vi "Get GEA3 COM Port.vi"(0 "GEA3 Serial Number":string, 11 "Error In":errorcluster) -> (4 "GEA3 COM Port":string, 15 "Error Out":errorcluster)   [LabVIEW 2016, in "GEA2_Toolkit.lvlib"]
uses:
  library/GEA2_Toolkit.lvlib
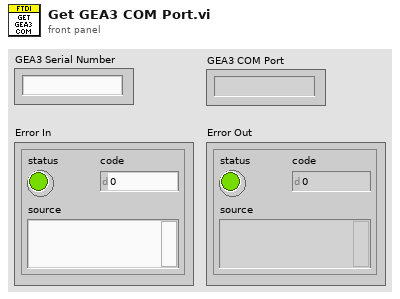
[diagram p1: front panel]
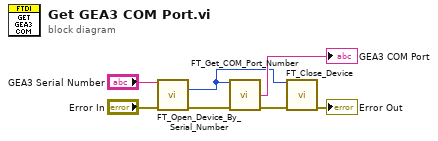
[diagram p0: block diagram]
diagram:
  n1 = call "FT_Open_Device_By_Serial_Number.vi"("Device Serial Number"="GEA3 Serial Number", "Error In"="Error In") -> ("Handle"=w4:u32, "Error Out"=w3:errorcluster)  [unwired: 11 in, 1 out]
  n2 = call "FT_Get_COM_Port_Number.vi"("Handle"=w4, "Error In"=w3) -> ("COM Port String"=→"GEA3 COM Port":string, "Error Out"=w5:errorcluster)  [unwired: 10 in, 2 out]
  n3 = call "FT_Close_Device.vi"("Handle"=w4, "Error In"=w5) -> ("Error Out"=→"Error Out":errorcluster)  [unwired: 12 in, 1 out]
